vi "solar_voy_def Export Value.vi"(0 "ID":bool, 1 "CMD":enum8{"CMD", "TLM"}(ring), 5 "SIZE":i32, 7 "TYPE":T1, 9 "EACH_SIZE (0=NoArray)":i32, 12 "MIN (NaN=Min)":dbl=nan, 13 "MAX (NaN=Max)":dbl=nan, 14 "DEFAULT (\"\"=Default)":string) -> (4 "VALUE_DEF":string)   [LabVIEW 2018]
doc: "This exports the parameter/item value to the COSMOS value fields depending on the type. If TYPE is INT, UINT or FLOAT this returns the MIN, MAX and VALUE. Otherwise only the VALUE is returned. Refer to: http://cosmosrb.com/docs/cmdtlm/"
uses:
  solar_voy_def_ctl ITEM TYPE.ctl
panel:
  out "Is Array?":bool
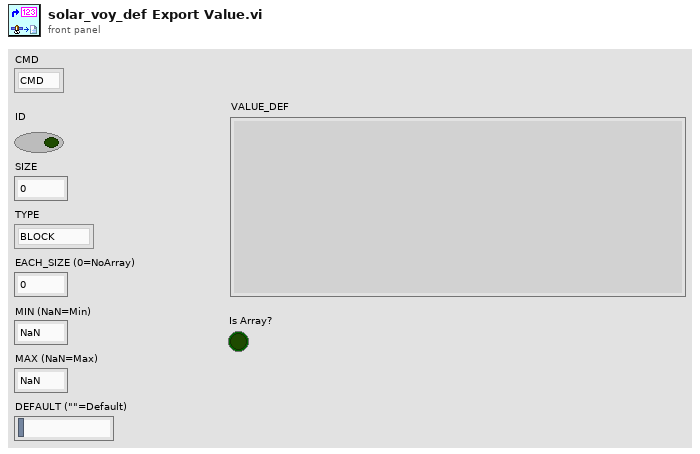
[diagram p1: front panel]
types:
  T1 = typedef "solar_voy_def_ctl ITEM TYPE.ctl" = enum8{"BLOCK", "INT", "UINT", "FLOAT", "STRING"}
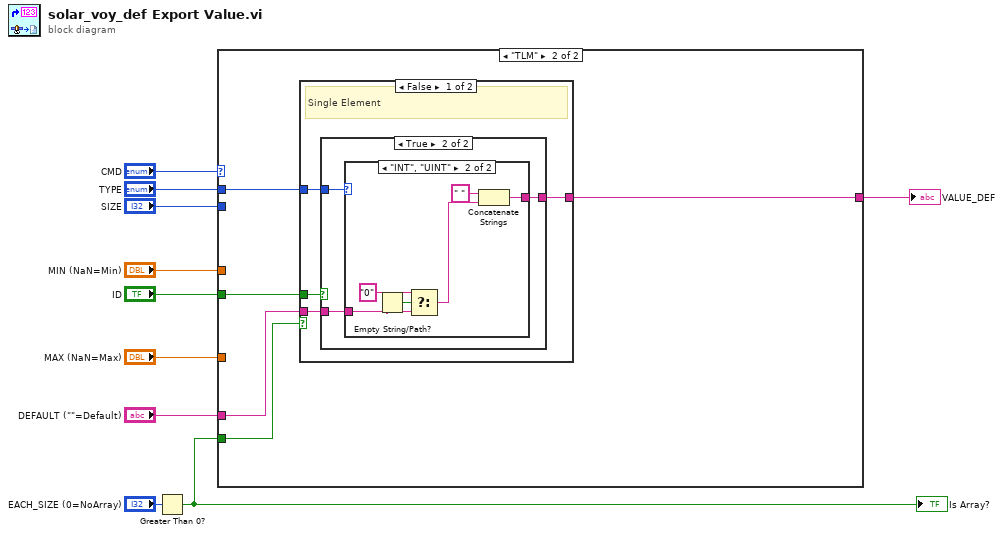
[diagram p0: block diagram]
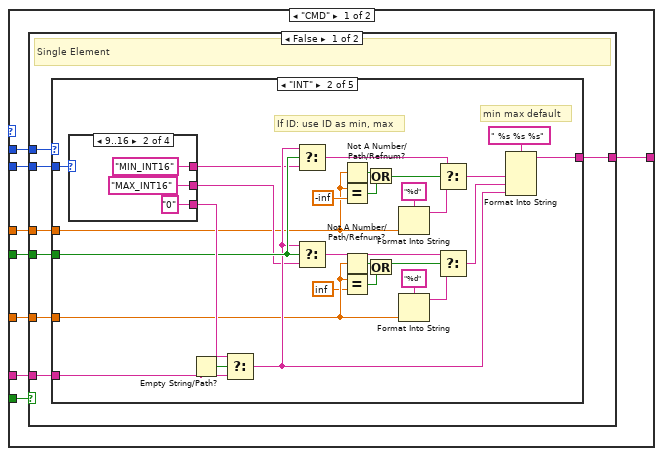
[diagram p2: hidden frame]
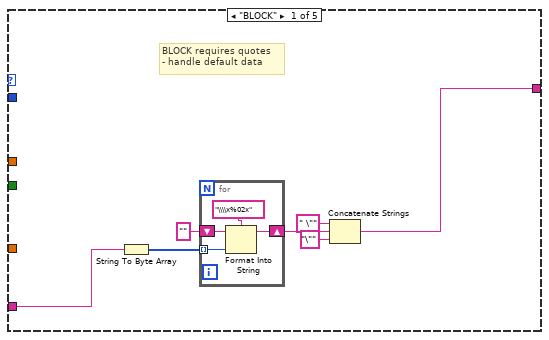
[diagram p3: hidden frame]
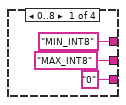
[diagram p4: hidden frame]
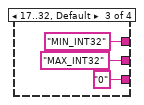
[diagram p5: hidden frame]
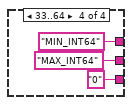
[diagram p6: hidden frame]
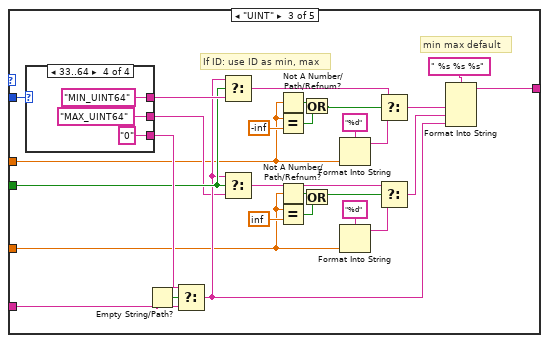
[diagram p7: hidden frame]
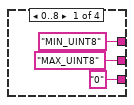
[diagram p8: hidden frame]
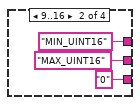
[diagram p9: hidden frame]
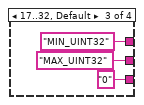
[diagram p10: hidden frame]
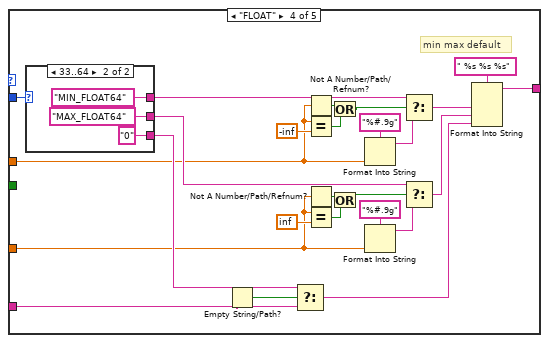
[diagram p11: hidden frame]
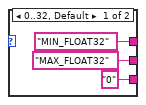
[diagram p12: hidden frame]
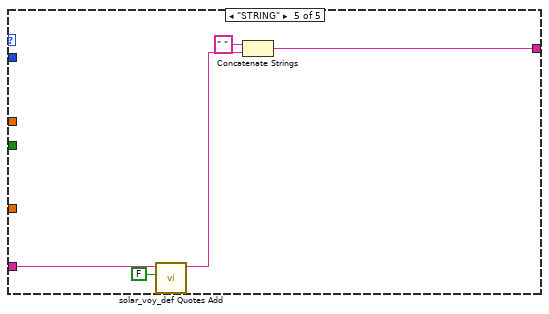
[diagram p13: hidden frame]
diagram:
  n1 = Greater Than 0?(x="EACH_SIZE (0=NoArray)") -> (x > 0?=w3:bool)
  "Is Array?" <- w3
  n2 = case shown="\"TLM\"" "CMD" {
    tunnel: "TYPE" -> [w18 w153]
    tunnel: "MIN (NaN=Min)" -> [w17 _]
    tunnel: "MAX (NaN=Max)" -> [w16 _]
    tunnel: "DEFAULT (\"\"=Default)" -> [w15 w156]
    tunnel: [w14 w155] -> w6
    tunnel: "SIZE" -> [w13 _]
    tunnel: w3 -> [w12 w154]
    tunnel: "ID" -> [w11 w157]
    frame "CMD" {
      n3 = case shown="False" w12 {
        tunnel: w18 -> [w25 _]
        tunnel: w17 -> [w24 _]
        tunnel: w16 -> [w23 _]
        tunnel: w15 -> [w22 _]
        tunnel: [w21 _] -> w14
        tunnel: w13 -> [w20 _]
        tunnel: w11 -> [w19 _]
        frame False {
          # "Single Element"
          n4 = case shown="\"INT\"" w25 {
            tunnel: w20 -> [_ w60 w102 w132 _]
            tunnel: w24 -> [_ w37 w77 w119 _]
            tunnel: w23 -> [_ w45 w78 w118 _]
            tunnel: w22 -> [w32 w57 w100 w128 w151]
            tunnel: [w26 w56 w99 w127 w149] -> w21
            tunnel: w19 -> [_ w51 w95 _ _]
            frame "BLOCK" {
              # "BLOCK requires quotes\n- handle default data"
              n5 = String To Byte Array(string=w32) -> (unsigned byte array=w31:u8[])
              n6 = for {
                tunnel: w31 -> [w36] mode=indexing
                shift-right: [w34] -> w29
                shift-left: "" -> [w33]
                n7 = Format Into String(format string="\\\\x%02x", initial string=w33, w36) -> (resulting string=w34:string)  [unwired: 1 in, 1 out]
              }
              n8 = Concatenate Strings(" \"", w29, "\"") -> (w26:string)
            }
            frame "INT" {
              # "If ID: use ID as min, max"
              # "min max default"
              n9 = case shown="9..16" w60 {
                tunnel: ["MIN_INT8" "MIN_INT16" "MIN_INT32" "MIN_INT64"] -> w46
                tunnel: ["MAX_INT8" "MAX_INT16" "MAX_INT32" "MAX_INT64"] -> w49
                tunnel: ["0" "0" "0" "0"] -> w62
                frame 0..8 {
                }
                frame 9..16 {
                }
                frame 17..32, Default {
                }
                frame 33..64 {
                }
              }
              n10 = Empty String/Path?(string/path=w57) -> (empty?=w63:bool)
              n11 = Select(t=w62, s=w63, f=w57) -> (s? t:f=w50:string)
              n12 = Select(t=w50, s=w51, f=w46) -> (s? t:f=w47:string)
              n13 = Select(t=w50, s=w51, f=w49) -> (s? t:f=w48:string)
              n14 = Not A Number/Path/Refnum?(number/path/refnum=w37) -> (NaN/Path/Refnum?=w39:bool)
              n15 = Equal?(x=w37, y=-inf) -> (x = y?=w41:bool)
              n16 = Not A Number/Path/Refnum?(number/path/refnum=w45) -> (NaN/Path/Refnum?=w64:bool)
              n17 = Equal?(x=w45, y=inf ("Positive Infinity")) -> (x = y?=w42:bool)
              n18 = Or(x=w39, y=w41) -> (x .or. y?=w38:bool)
              n19 = Or(x=w64, y=w42) -> (x .or. y?=w43:bool)
              n20 = Format Into String(format string="%d", w37) -> (resulting string=w53:string)  [unwired: 2 in, 1 out]
              n21 = Format Into String(format string="%d", w45) -> (resulting string=w54:string)  [unwired: 2 in, 1 out]
              n22 = Select(t=w47, s=w38, f=w53) -> (s? t:f=w61:string)
              n23 = Select(t=w48, s=w43, f=w54) -> (s? t:f=w58:string)
              n24 = Format Into String(format string=" %s %s %s", w61, w58, w50) -> (resulting string=w56:string)  [unwired: 2 in, 1 out]
            }
            frame "UINT" {
              # "If ID: use ID as min, max"
              # "min max default"
              n25 = case shown="33..64" w102 {
                tunnel: ["MIN_UINT8" "MIN_UINT16" "MIN_UINT32" "MIN_UINT64"] -> w96
                tunnel: ["MAX_UINT8" "MAX_UINT16" "MAX_UINT32" "MAX_UINT64"] -> w87
                tunnel: ["0" "0" "0" "0"] -> w103
                frame 0..8 {
                }
                frame 9..16 {
                }
                frame 17..32, Default {
                }
                frame 33..64 {
                }
              }
              n26 = Empty String/Path?(string/path=w100) -> (empty?=w104:bool)
              n27 = Select(t=w103, s=w104, f=w100) -> (s? t:f=w94:string)
              n28 = Select(t=w94, s=w95, f=w96) -> (s? t:f=w89:string)
              n29 = Select(t=w94, s=w95, f=w87) -> (s? t:f=w88:string)
              n30 = Not A Number/Path/Refnum?(number/path/refnum=w77) -> (NaN/Path/Refnum?=w81:bool)
              n31 = Equal?(x=w77, y=-inf) -> (x = y?=w83:bool)
              n32 = Not A Number/Path/Refnum?(number/path/refnum=w78) -> (NaN/Path/Refnum?=w86:bool)
              n33 = Equal?(x=w78, y=inf ("Positive Infinity")) -> (x = y?=w84:bool)
              n34 = Or(x=w81, y=w83) -> (x .or. y?=w80:bool)
              n35 = Or(x=w86, y=w84) -> (x .or. y?=w79:bool)
              n36 = Format Into String(format string="%d", w77) -> (resulting string=w91:string)  [unwired: 2 in, 1 out]
              n37 = Format Into String(format string="%d", w78) -> (resulting string=w92:string)  [unwired: 2 in, 1 out]
              n38 = Select(t=w89, s=w80, f=w91) -> (s? t:f=w97:string)
              n39 = Select(t=w88, s=w79, f=w92) -> (s? t:f=w98:string)
              n40 = Format Into String(format string=" %s %s %s", w97, w98, w94) -> (resulting string=w99:string)  [unwired: 2 in, 1 out]
            }
            frame "FLOAT" {
              # "min max default"
              n41 = case shown="33..64" w132 {
                tunnel: ["MIN_FLOAT32" "MIN_FLOAT64"] -> w137
                tunnel: ["MAX_FLOAT32" "MAX_FLOAT64"] -> w136
                tunnel: ["0" "0"] -> w134
                frame 0..32, Default {
                }
                frame 33..64 {
                }
              }
              n42 = Empty String/Path?(string/path=w128) -> (empty?=w135:bool)
              n43 = Select(t=w134, s=w135, f=w128) -> (s? t:f=w129:string)
              n44 = Not A Number/Path/Refnum?(number/path/refnum=w119) -> (NaN/Path/Refnum?=w121:bool)
              n45 = Equal?(x=w119, y=-inf) -> (x = y?=w123:bool)
              n46 = Not A Number/Path/Refnum?(number/path/refnum=w118) -> (NaN/Path/Refnum?=w126:bool)
              n47 = Equal?(x=w118, y=inf ("Positive Infinity")) -> (x = y?=w124:bool)
              n48 = Or(x=w121, y=w123) -> (x .or. y?=w120:bool)
              n49 = Or(x=w126, y=w124) -> (x .or. y?=w117:bool)
              n50 = Format Into String(format string="%#.9g", w119) -> (resulting string=w139:string)  [unwired: 2 in, 1 out]
              n51 = Format Into String(format string="%#.9g", w118) -> (resulting string=w140:string)  [unwired: 2 in, 1 out]
              n52 = Select(t=w137, s=w120, f=w139) -> (s? t:f=w133:string)
              n53 = Select(t=w136, s=w117, f=w140) -> (s? t:f=w130:string)
              n54 = Format Into String(format string=" %s %s %s", w133, w130, w129) -> (resulting string=w127:string)  [unwired: 2 in, 1 out]
            }
            frame "STRING" {
              n55 = call "solar_voy_def Quotes Add.vi"("Whitespace Only? (F=Always)"=FALSE, "String"=w151) -> ("String with Comments"=w150:string)  [unwired: 9 in]
              n56 = Concatenate Strings(" " ("string"), w150) -> (w149:string)
            }
          }
        }
        frame True {
          # "Array of Elements\n-no min, max, default"
        }
      }
    }
    frame "TLM" {
      n57 = case shown="False" w154 {
        tunnel: w157 -> [w161 _]
        tunnel: w156 -> [w160 _]
        tunnel: [w159 _] -> w155
        tunnel: w153 -> [w158 _]
        frame False {
          # "Single Element"
          n58 = case shown="True" w161 {
            tunnel: w160 -> [_ w164]
            tunnel: [_ w163] -> w159
            tunnel: w158 -> [_ w162]
            frame False {
            }
            frame True {
              n59 = case shown="\"INT\", \"UINT\"" w162 {
                tunnel: w164 -> [_ w169]
                tunnel: [_ w166] -> w163
                frame "BLOCK", "FLOAT", "STRING" {
                }
                frame "INT", "UINT" {
                  n60 = Empty String/Path?(string/path=w169) -> (empty?=w170:bool)
                  n61 = Select(t="0", s=w170, f=w169) -> (s? t:f=w167:string)
                  n62 = Concatenate Strings(" " ("string"), w167) -> (w166:string)
                }
              }
            }
          }
        }
        frame True {
          # "Array of Elements\n-no IDs"
        }
      }
    }
  }
  "VALUE_DEF" <- w6
